vi "线性公式.vi"(0 "标液浓度":dbl[](array[numeric]), 1 "信号值":dbl[](array[numeric]), 4 "启用":bool[](array[boolean]), 5 "method":T1 caption="方法" items=["最小二乘", "最小绝对残差", "Bisquare"], 6 "模型":enum32{"线性", "多项式", "折线"}(ring), 7 "精度":i32=6) -> (13 "Polynomial Coefficients 2":dbl[](array[numeric]) caption="多项式系数2", 14 "拟合方程":string, 15 "r^2":dbl format="%.7g", 16 "拟合方程 2":string, 17 "r^2 2":dbl caption="r^2" format="%.7g", 18 "XY图":cluster{"X Values":dbl[], "Y Values":dbl[]}[](graph), 19 "Polynomial Coefficients":dbl[](array[numeric]) caption="多项式系数")   [LabVIEW 2016, in "斯坦道原位多参数.lvlib"]
uses:
  <vilib>/Analysis/6fits.llb/Curve Fitting Criteria.ctl
  <vilib>/Analysis/NI_AALPro.lvlib
  <vilib>/gmath/NI_Gmath.lvlib
panel:
  out "Best Linear Fit 2":dbl[](array[numeric]) caption="最佳线性拟合2"
  out "Best Linear Fit":dbl[](array[numeric]) caption="最佳线性拟合"
  out "二维数组":dbl[][](array[numeric])
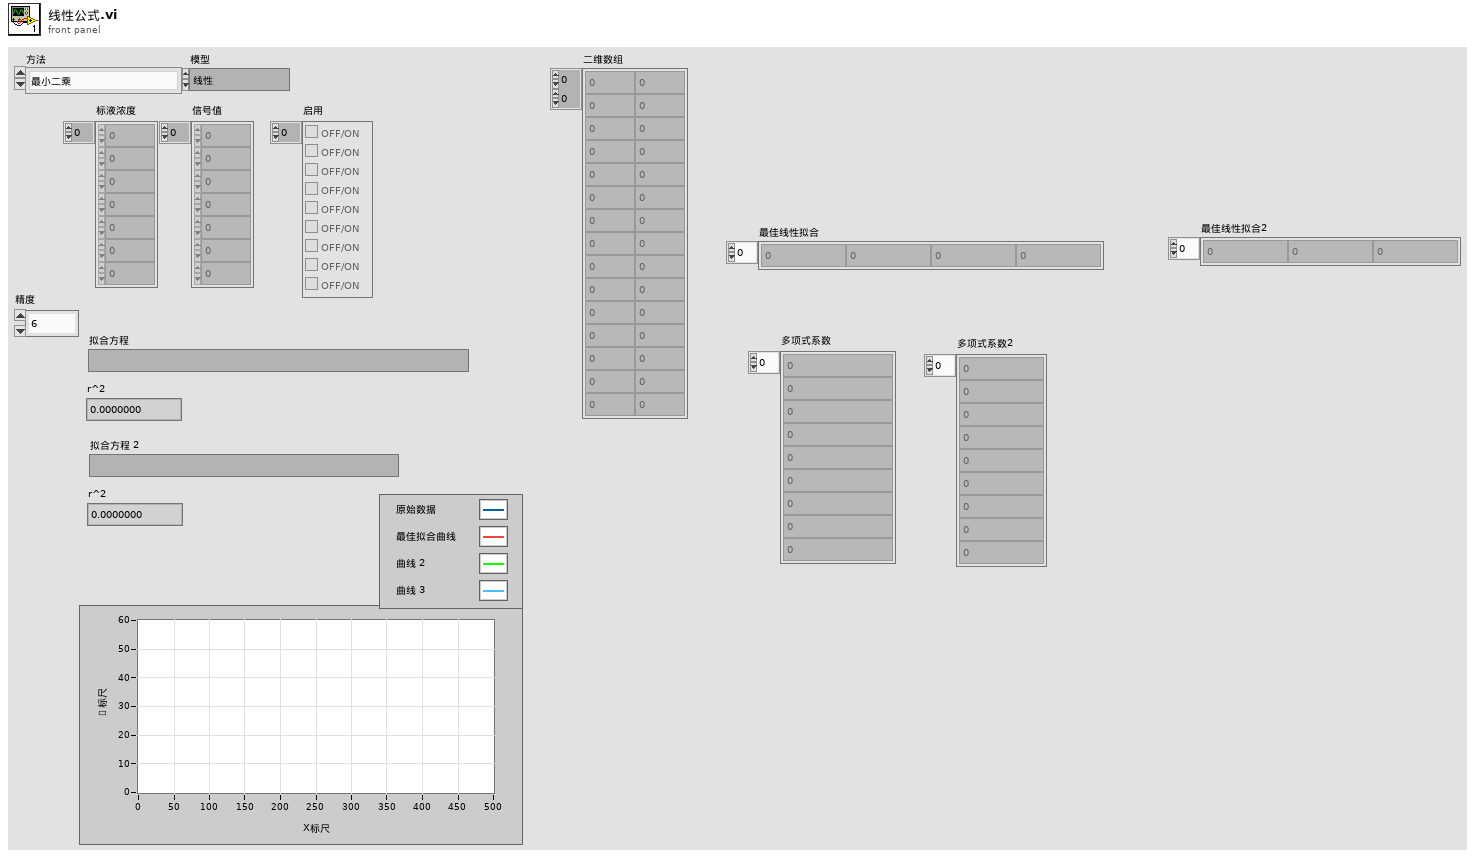
[diagram p1: front panel]
types:
  T1 = typedef "NI_AALPro.lvlib/Curve Fitting Criteria.ctl" = u16
  T2 = enum16{"Linear", "Polynomial", "Exponential", "Power"}
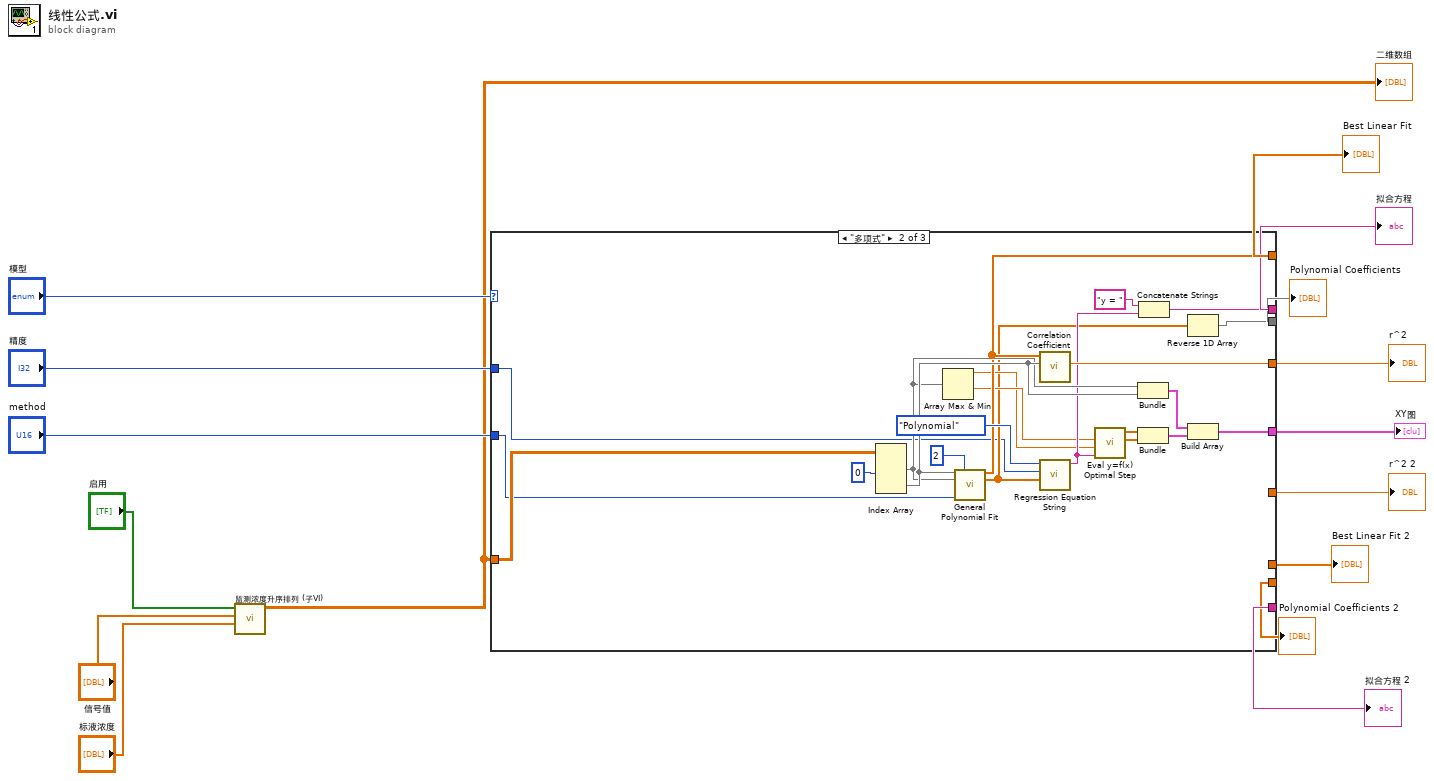
[diagram p0: block diagram]
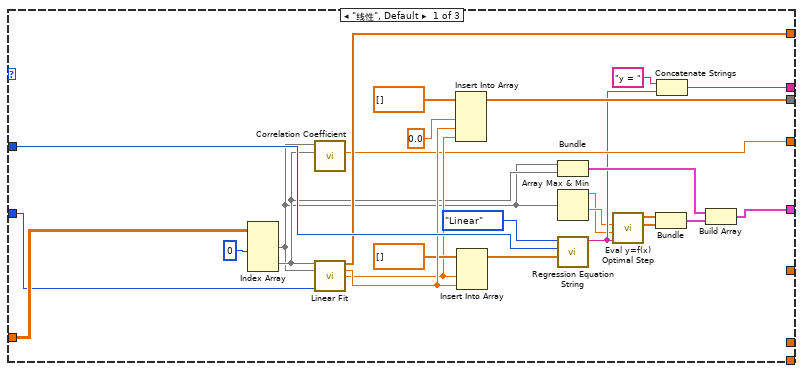
[diagram p2: hidden frame]
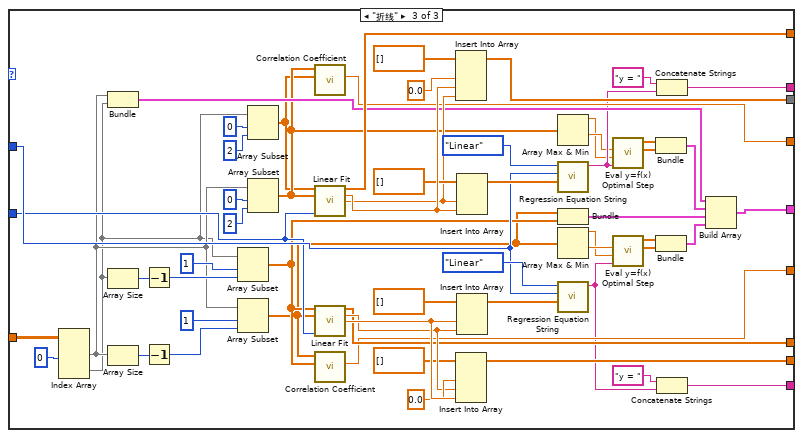
[diagram p3: hidden frame]
diagram:
  n1 = call "监测浓度升序排列 (子VI).vi"("标液浓度"="标液浓度", "滴定数"="信号值", "启用"="启用") -> ("输出数组"=w1:dbl[][])  [unwired: 8 in]
  "二维数组" <- w1
  n2 = case shown="\"多项式\"" "模型" {
    tunnel: w1 -> [w41 w57 w112]
    tunnel: "精度" -> [w34 w43 w90]
    tunnel: [w28 w48 w109] -> w11
    tunnel: [w27 w52 w108] -> w10
    tunnel: [w26 w55 w110] -> w9
    tunnel: [w25 w56 w111] -> w8
    tunnel: [w23 w53 w107] -> w7
    tunnel: "method" -> [w20 w49 w89]
    tunnel: [_ _ w94] -> w5
    tunnel: [_ _ w93] -> w4
    tunnel: [_ _ w92] -> w3
    tunnel: [_ _ w91] -> w2
    frame "线性", Default {
      n3 = Index Array(array=w41, index (col) #1=0 ("禁用的索引 (列)")) -> (element #1=w21:dbl[], element #2=w22:dbl[])  [unwired: 3 in]
      n4 = call <vilib>:"Correlation Coefficient.vi"("Y"=w22, "X"=w21) -> ("r^2"=w27:dbl)  [unwired: 8 in, 1 out]
      n5 = call <vilib>:"Linear Fit.vi"("Y"=w22, "X"=w21, "method"=w20) -> ("Best Linear Fit"=w28:dbl[], "slope"=w32:dbl, "intercept"=w29:dbl)  [unwired: 8 in, 2 out]
      n6 = Insert Into Array(array=dbl[] [] ("数组"), new element #1=0.0 ("新元素/子数组"), new element #2=w32, new element #3=w29) -> (w23:dbl[])  [unwired: 1 in]
      n7 = Insert Into Array(array=dbl[] [] ("数组"), new element #1=w29, new element #2=w32) -> (w24:dbl[])  [unwired: 1 in]
      n8 = Bundle("输出数组"=w21, "输出数组"=w22) -> (w38:cluster{"输出数组":dbl[], "输出数组":dbl[]})  [unwired: 1 in]
      n9 = Array Max & Min(array=w21) -> (max value=w17:dbl, min value=w18:dbl)  [unwired: 2 out]
      n10 = call "Regression Equation String.vi"("系数"=w24, "精度"=w34, "拟合类型"=T2."Linear") -> ("公式"=w19:string)  [unwired: 8 in]
      n11 = call <vilib>:"Eval y=f(x) Optimal Step.vi"("formula"=w19, "end"=w17, "start"=w18) -> ("Y Values"=w40:dbl[], "X Values"=w39:dbl[])  [unwired: 2 in, 2 out]
      n12 = Bundle("X Values"=w39, "Y Values"=w40) -> (w37:cluster{"X Values":dbl[], "Y Values":dbl[]})  [unwired: 1 in]
      n13 = Concatenate Strings("y = " ("string"), w19) -> (w26:string)
      n14 = Build Array(w38, w37) -> (w25:cluster{"X Values":dbl[], "Y Values":dbl[]}[])
    }
    frame "多项式" {
      n15 = Index Array(array=w57, index (col) #1=0 ("禁用的索引 (列)")) -> (element #1=w50:dbl[], element #2=w51:dbl[])  [unwired: 3 in]
      n16 = Array Max & Min(array=w50) -> (max value=w45:dbl, min value=w46:dbl)  [unwired: 2 out]
      n17 = call <vilib>:"General Polynomial Fit.vi"("Y"=w51, "polynomial order"=2, "X"=w50, "method"=w49) -> ("Best Polynomial Fit"=w48:dbl[], "Polynomial Coefficients"=w44:dbl[])  [unwired: 8 in, 2 out]
      n18 = call <vilib>:"Correlation Coefficient.vi"("Y"=w51, "X"=w48) -> ("r^2"=w52:dbl)  [unwired: 8 in, 1 out]
      n19 = call "Regression Equation String.vi"("系数"=w44, "精度"=w43, "拟合类型"=T2."Polynomial") -> ("公式"=w47:string)  [unwired: 8 in]
      n20 = call <vilib>:"Eval y=f(x) Optimal Step.vi"("formula"=w47, "end"=w45, "start"=w46) -> ("Y Values"=w63:dbl[], "X Values"=w62:dbl[])  [unwired: 2 in, 2 out]
      n21 = Bundle("输出数组"=w50, "输出数组"=w51) -> (w61:cluster{"输出数组":dbl[], "输出数组":dbl[]})  [unwired: 1 in]
      n22 = Bundle("X Values"=w62, "Y Values"=w63) -> (w60:cluster{"X Values":dbl[], "Y Values":dbl[]})  [unwired: 1 in]
      n23 = Concatenate Strings("y = " ("string"), w47) -> (w55:string)
      n24 = Reverse 1D Array(array=w44) -> (reversed array=w53:dbl[])
      n25 = Build Array(w61, w60) -> (w56:cluster{"X Values":dbl[], "Y Values":dbl[]}[])
    }
    frame "折线" {
      n26 = Index Array(array=w112, index (col) #1=0 ("禁用的索引 (列)")) -> (element #1=w66:dbl[], element #2=w65:dbl[])  [unwired: 3 in]
      n27 = Bundle("输出数组"=w66, "输出数组"=w65) -> (w82:cluster{"输出数组":dbl[], "输出数组":dbl[]})  [unwired: 1 in]
      n28 = Array Size(array=w65) -> (size(s)=w87:i32)
      n29 = Array Size(array=w66) -> (size(s)=w85:i32)
      n30 = Decrement(x=w87) -> (x-1=w86:i32)
      n31 = Decrement(x=w85) -> (x-1=w83:i32)
      n32 = Array Subset(array=w65, index=1 ("索引"), length=w86) -> (w81:dbl[])
      n33 = Array Subset(array=w66, index=1 ("索引"), length=w83) -> (w74:dbl[])
      n34 = Array Subset(array=w65, index=0 ("索引"), length=2 ("长度")) -> (w71:dbl[])
      n35 = Array Subset(array=w66, index=0 ("索引"), length=2 ("长度")) -> (w72:dbl[])
      n36 = call <vilib>:"Correlation Coefficient.vi"("Y"=w71, "X"=w72) -> ("r^2"=w108:dbl)  [unwired: 8 in, 1 out]
      n37 = call <vilib>:"Linear Fit.vi"("Y"=w71, "X"=w72, "method"=w89) -> ("Best Linear Fit"=w109:dbl[], "slope"=w117:dbl, "intercept"=w114:dbl)  [unwired: 8 in, 2 out]
      n38 = call <vilib>:"Linear Fit.vi"("Y"=w81, "X"=w74, "method"=w89) -> ("Best Linear Fit"=w94:dbl[], "slope"=w98:dbl, "intercept"=w101:dbl)  [unwired: 8 in, 2 out]
      n39 = call <vilib>:"Correlation Coefficient.vi"("Y"=w81, "X"=w74) -> ("r^2"=w93:dbl)  [unwired: 8 in, 1 out]
      n40 = Insert Into Array(array=dbl[] [] ("数组"), new element #1=0.0 ("新元素/子数组"), new element #2=w117, new element #3=w114) -> (w107:dbl[])  [unwired: 1 in]
      n41 = Insert Into Array(array=dbl[] [] ("数组"), new element #1=0.0 ("新元素/子数组"), new element #2=w98, new element #3=w101) -> (w91:dbl[])  [unwired: 1 in]
      n42 = Insert Into Array(array=dbl[] [] ("数组"), new element #1=w114, new element #2=w117) -> (w113:dbl[])  [unwired: 1 in]
      n43 = Insert Into Array(array=dbl[] [] ("数组"), new element #1=w101, new element #2=w98) -> (w102:dbl[])  [unwired: 1 in]
      n44 = Array Max & Min(array=w72) -> (max value=w69:dbl, min value=w70:dbl)  [unwired: 2 out]
      n45 = call "Regression Equation String.vi"("系数"=w113, "精度"=w90, "拟合类型"=T2."Linear") -> ("公式"=w80:string)  [unwired: 8 in]
      n46 = Bundle(w74, w81) -> (w75:cluster{dbl[], dbl[]})  [unwired: 1 in]
      n47 = Array Max & Min(array=w74) -> (max value=w67:dbl, min value=w68:dbl)  [unwired: 2 out]
      n48 = call "Regression Equation String.vi"("系数"=w102, "精度"=w90, "拟合类型"=T2."Linear") -> ("公式"=w73:string)  [unwired: 8 in]
      n49 = call <vilib>:"Eval y=f(x) Optimal Step.vi"("formula"=w80, "end"=w69, "start"=w70) -> ("Y Values"=w122:dbl[], "X Values"=w121:dbl[])  [unwired: 2 in, 2 out]
      n50 = call <vilib>:"Eval y=f(x) Optimal Step.vi"("formula"=w73, "end"=w67, "start"=w68) -> ("Y Values"=w78:dbl[], "X Values"=w79:dbl[])  [unwired: 2 in, 2 out]
      n51 = Bundle("X Values"=w121, "Y Values"=w122) -> (w76:cluster{"X Values":dbl[], "Y Values":dbl[]})  [unwired: 1 in]
      n52 = Bundle("X Values"=w79, "Y Values"=w78) -> (w77:cluster{"X Values":dbl[], "Y Values":dbl[]})  [unwired: 1 in]
      n53 = Concatenate Strings("y = " ("string"), w80) -> (w110:string)
      n54 = Concatenate Strings("y = " ("string"), w73) -> (w92:string)
      n55 = Build Array(w82, w76, w75, w77) -> (w111:cluster{"X Values":dbl[], "Y Values":dbl[]}[])
    }
  }
  "Best Linear Fit" <- w11
  "r^2" <- w10
  "拟合方程" <- w9
  "XY图" <- w8
  "Polynomial Coefficients" <- w7
  "r^2 2" <- w4
  "拟合方程 2" <- w3
  "Best Linear Fit 2" <- w5
  "Polynomial Coefficients 2" <- w2
